vi "Configure Scan.vi"(0 "VISA resource name":refnum<visa-resource-name>, 1 "Scan Mode (0: None)":u16(ring) items=["None", "Internal", "External"], 2 "Starting Channel (1)":i32=1, 3 "Stopping Channel (10)":i32=10, 5 "error in (no error)":errorcluster) -> (14 "VISA resource name out":refnum<visa-resource-name>, 19 "error out":errorcluster)   [LabVIEW 2013, in "Keithley 2000.lvlib"]
doc: "This VI configures the scanning operation of the instrument. This VI is only valid if you have an internal or external scanner card."
uses:
  Keithley 2000.lvlib
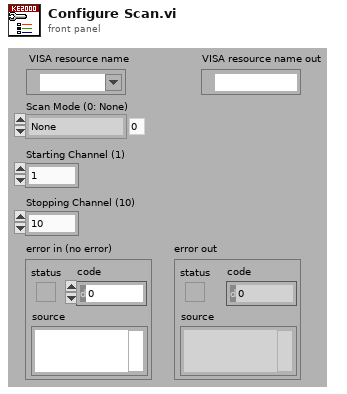
[diagram p1: front panel]
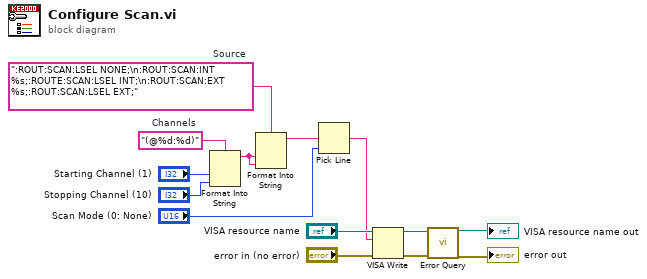
[diagram p0: block diagram]
diagram:
  w9 = ":ROUT:SCAN:LSEL NONE;\n:ROUT:SCAN:INT %s;:ROUTE:SCAN:LSEL INT;\n:ROUT:SCAN:EXT %s;:ROUT:SCAN:LSEL EXT;"  # Source
  w12 = "(@%d:%d)"  # Channels
  n1 = Format Into String(format string=w12, "Starting Channel (1)", "Stopping Channel (10)") -> (resulting string=w8:string)  [unwired: 2 in, 1 out]
  n2 = Format Into String(format string=w9, w8, w8) -> (resulting string=w7:string)  [unwired: 2 in, 1 out]
  n3 = Pick Line(multi-line string=w7, line index="Scan Mode (0: None)") -> (output string=w5:string)  [unwired: 1 in]
  n4 = VISA Write(VISA resource name="VISA resource name", write buffer=w5, error in (no error)="error in (no error)") -> (VISA resource name out=w4:refnum<visa-resource-name>, error out=w3:errorcluster)  [unwired: 1 out]
  n5 = call "Error Query.vi"("VISA resource name"=w4, "error in (no error)"=w3) -> ("VISA resource name out"=→"VISA resource name out":refnum<visa-resource-name>, "error out"=→"error out":errorcluster)  [unwired: 14 in, 2 out]
